vi "RCstage_Test_MV.vi"(2 "error in":errorcluster, 3 "Pos. Index":i32, 4 "Stage Ref. In":refnum<visa-resource-name>) -> (0 "error out":errorcluster={"status"=FALSE, "code"=1073676418, "source"="VISA Close in RCstage_Test.vi"}, 1 "Stage Ref. Out":refnum<visa-resource-name>)   [LabVIEW 2017]
panel:
  out "Command out":string=":0106980000025F\r\n"
  # "Stage Move: Index 0 is safety position"
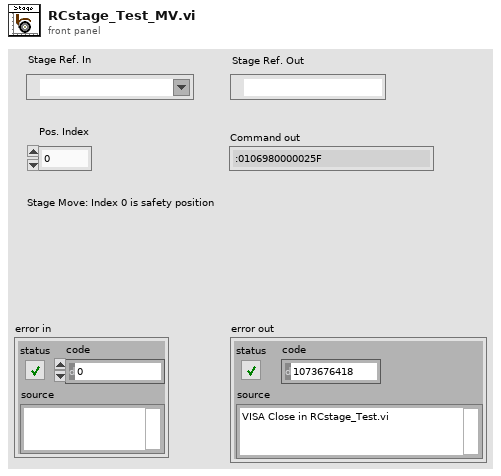
[diagram p1: front panel]
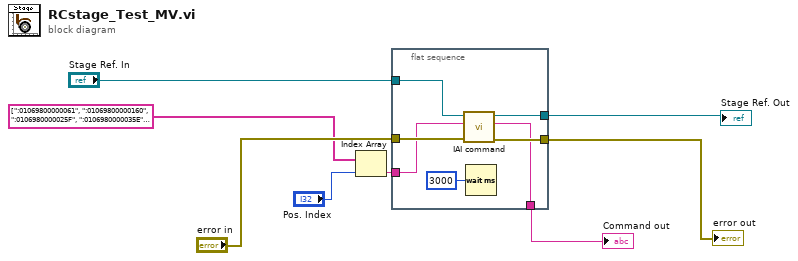
[diagram p0: block diagram]
diagram:
  n1 = Index Array(array=string[] [":01069800000061", ":01069800000160", ":0106980000025F", ":0106980000035E", ":0106980000045D", ":0106980000055C", ":0106980000065B", ":0106980000075A", ":01069800000859", ":01069800000958", ":01069800000A57", ":01069800000B56", ":01069800000C55", ":01069800000D54", ":01069800000E53", ":01069800000F52"] ("Stage_Command"), index="Pos. Index") -> (element=w4:string)
  n2 = flat-sequence {
    tunnel: [w15] -> w8
    tunnel: [w14] -> w7
    tunnel: "error in" -> [w13]
    tunnel: "Stage Ref. In" -> [w12]
    tunnel: w4 -> [w10]
    tunnel: [w9] -> w3
    frame #0 {
      n3 = call "IAI command.vi"("error in (no error)"=w13, "packet"=w10, "VISA Refnum in"=w12) -> ("error out"=w14:errorcluster, "read buffer"=w9:string, "VISA Refnum"=w15:refnum<visa-resource-name>)  [unwired: 6 in]
      n4 = Wait (ms)(milliseconds to wait=u32 3000) -> ()  [unwired: 1 out]
    }
  }
  "error out" <- w7
  "Stage Ref. Out" <- w8
  "Command out" <- w3
